vi "LinearInterpolate.vi"(10 "Config":T1, 11 "Value":dbl) -> (3 "Ouput":dbl)   [LabVIEW 2016]
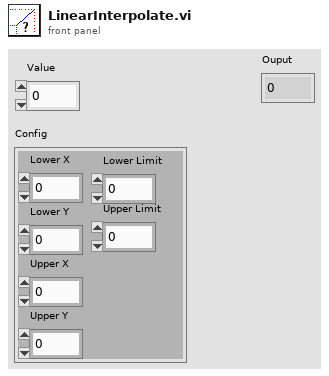
[diagram p1: front panel]
types:
  T1 = cluster{"Lower X":dbl, "Lower Y":dbl, "Upper X":dbl, "Upper Y":dbl, "Lower Limit":dbl, "Upper Limit":dbl}
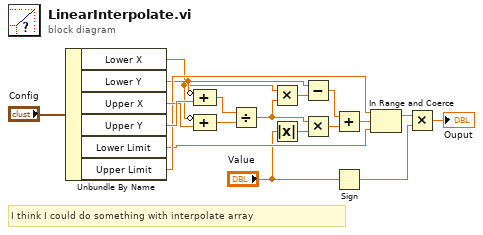
[diagram p0: block diagram]
diagram:
  # "I think I could do something with interpolate array"
  n1 = Unbundle By Name("Config") -> ("Lower X"=w8:dbl, "Lower Y"=w10:dbl, "Upper X"=w17:dbl, "Upper Y"=w18:dbl, "Lower Limit"=w13:dbl, "Upper Limit"=w14:dbl)
  n2 = Compound Arithmetic op=ADD(invert w10, w18) -> (w16:dbl)
  n3 = Compound Arithmetic op=ADD(invert w8, w17) -> (w15:dbl)
  n4 = Divide(x=w16, y=w15) -> (x/y=w9:dbl)
  n5 = Multiply(x=w8, y=w9) -> (x*y=w7:dbl)
  n6 = Absolute Value(x="Value") -> (abs(x)=w5:dbl)
  n7 = Subtract(x=w10, y=w7) -> (x-y=w6:dbl)
  n8 = Multiply(x=w9, y=w5) -> (x*y=w12:dbl)
  n9 = Add(x=w6, y=w12) -> (x+y=w11:dbl)
  n10 = Sign(1:"Value") -> (0:w2:dbl)
  n11 = In Range and Coerce(upper limit=w14, x=w11, lower limit=w13) -> (coerced(x)=w4:dbl)  [unwired: 1 out]
  n12 = Multiply(x=w4, y=w2) -> (x*y=→"Ouput":dbl)
